vi "Update Class Wire Appearance.vi"(8 "error in (no error)":errorcluster, 9 "UI Color":u32(colorbox), 10 "Color":u32(colorbox), 11 "ProjectItem in":refnum<class "ProjectItem.lvclass">) -> (0 "error out":errorcluster, 3 "ProjectItem out":refnum<class "ProjectItem.lvclass">)   [LabVIEW 2019, in "ProjectItem.lvclass"]
uses:
  ProjectItem.lvclass
  ProjectItem.lvclass/ProjectItem.ctl
panel:
  out "Class Names":string[](array[string])
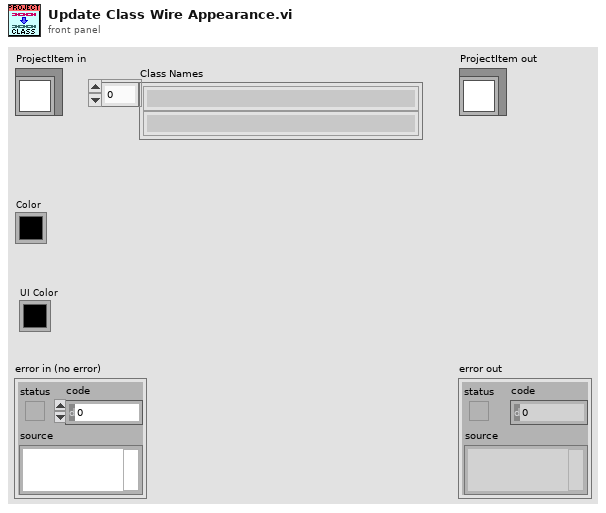
[diagram p1: front panel]
types:
  T1 = cluster{"Class":refnum<vi>, "DynamicVIs":refnum<vi>[], "StaticVIs":refnum<vi>[], "Controls":refnum<vi>[], "Name":string, "Icon":refnum<class "Icon.lvclass">, "Wire Foreground Color":u32}[]
  T2 = cluster{"Foreground Color":u32, "Background Color":u32, "Fill Pattern":cluster{"Row 0":u8, "Row 1":u8, "Row 2":u8, "Row 3":u8, "Row 4":u8, "Row 5":u8, "Row 6":u8, "Row 7":u8}, "Width":i16, "Mode":enum16{"Copy", "Or", "Exclusive Or", "Bit Clear", "Not Copy", "Not Or", "Nor Exclusive Or", "Not Bit Clear"}, "Style":enum32{"Solid", "Dash", "Dot", "Dash Dot", "Dash Dot Dot"}, "Fill Rule":enum32{"Even Odd", "Winding"}, "End Caps":enum32{"Default", "Flat"}}[]
  T3 = cluster{"Foreground Color":u32, "Background Color":u32, "Fill Pattern":cluster{"Row 0":u8, "Row 1":u8, "Row 2":u8, "Row 3":u8, "Row 4":u8, "Row 5":u8, "Row 6":u8, "Row 7":u8}, "Width":i16, "Mode":enum16{"Copy", "Or", "Exclusive Or", "Bit Clear", "Not Copy", "Not Or", "Nor Exclusive Or", "Not Bit Clear"}, "Style":enum32{"Solid", "Dash", "Dot", "Dash Dot", "Dash Dot Dot"}, "Fill Rule":enum32{"Even Odd", "Winding"}, "End Caps":enum32{"Default", "Flat"}}
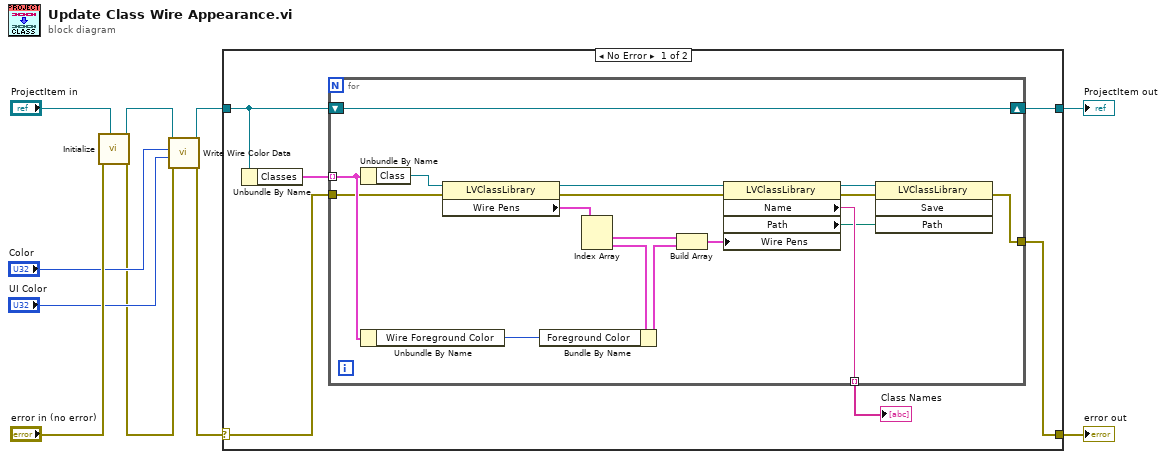
[diagram p0: block diagram]
diagram:
  n1 = call "Initialize.vi"("ProjectItem"="ProjectItem in", "error in (no error)"="error in (no error)") -> ("error out"=w2:errorcluster, "ProjectItem out"=w4:refnum<class "ProjectItem.lvclass">)  [unwired: 8 in]
  n2 = call "Write Wire Color Data.vi"("error in (no error)"=w2, "UI Color"="UI Color", "Color"="Color", "ProjectItem in"=w4) -> ("error out"=w1:errorcluster, "ProjectItem out"=w3:refnum<class "ProjectItem.lvclass">)  [unwired: 6 in]
  n3 = case shown="No Error" w1 {
    selector: w1 -> [w12 w35]
    tunnel: [w16 w35] -> w10
    tunnel: [w15 w34] -> w9
    tunnel: w3 -> [w13 w34]
    frame No Error {
      n4 = Unbundle By Name(w13) -> ("Classes"=w14:T1)
      n5 = for {
        tunnel: [w30] -> w16
        tunnel: [w32] -> w11 mode=indexing
        tunnel: w14 -> [w23] mode=indexing
        tunnel: w12 -> [w19]
        shift-right: [w31] -> w15
        shift-left: w13 -> [w31]
        n6 = Unbundle By Name(w23) -> ("Class"=w22:refnum<vi>)
        n7 = Unbundle By Name(w23) -> ("Wire Foreground Color"=w17:u32)
        n8 = property class="LVClassLibrary"(reference=w22, error in=w19) -> (reference out=w21:refnum<vi>, error out=w20:errorcluster, "Wire Pens"=w18:T2)
        n9 = Index Array(array=w18) -> (element #1=w26:T3, element #2=w28:T3)  [unwired: 2 in]
        n10 = Bundle By Name(cluster=w28, "Foreground Color"=w17) -> (w27:T3)
        n11 = Build Array(w26, w27) -> (w24:T2)
        n12 = property class="LVClassLibrary"(reference=w21, error in=w20, "Wire Pens"=w24) -> (reference out=w33:refnum<vi>, error out=w29:errorcluster, "Name"=w32:string, "Path"=w25:path)
        n13 = invoke class="LVClassLibrary" method="Save"(reference=w33, error in=w29, "Path"=w25) -> (error out=w30:errorcluster)  [unwired: 1 in, 3 out]
      }
      "Class Names" <- w11
    }
    frame Error {
    }
  }
  "error out" <- w10
  "ProjectItem out" <- w9
